vi "ISO226.vi"(11 "Phone number":dbl=1.0) -> (2 "SPL":dbl[](array[numeric]), 3 "Frequency":dbl[](array[numeric]))   [LabVIEW 2013]
uses:
  Stimulus/SubVI/CRYStimulus Global.vi
panel:
  out "XY Graph":cluster{dbl[], dbl[]}(graph)
  out "f":dbl[](array[numeric])
  in  "step number":i32=29
  in  "Resolution":u16
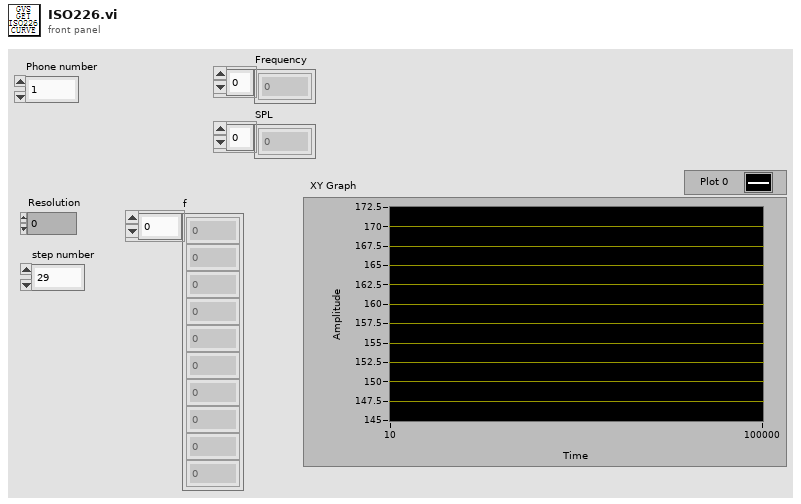
[diagram p1: front panel]
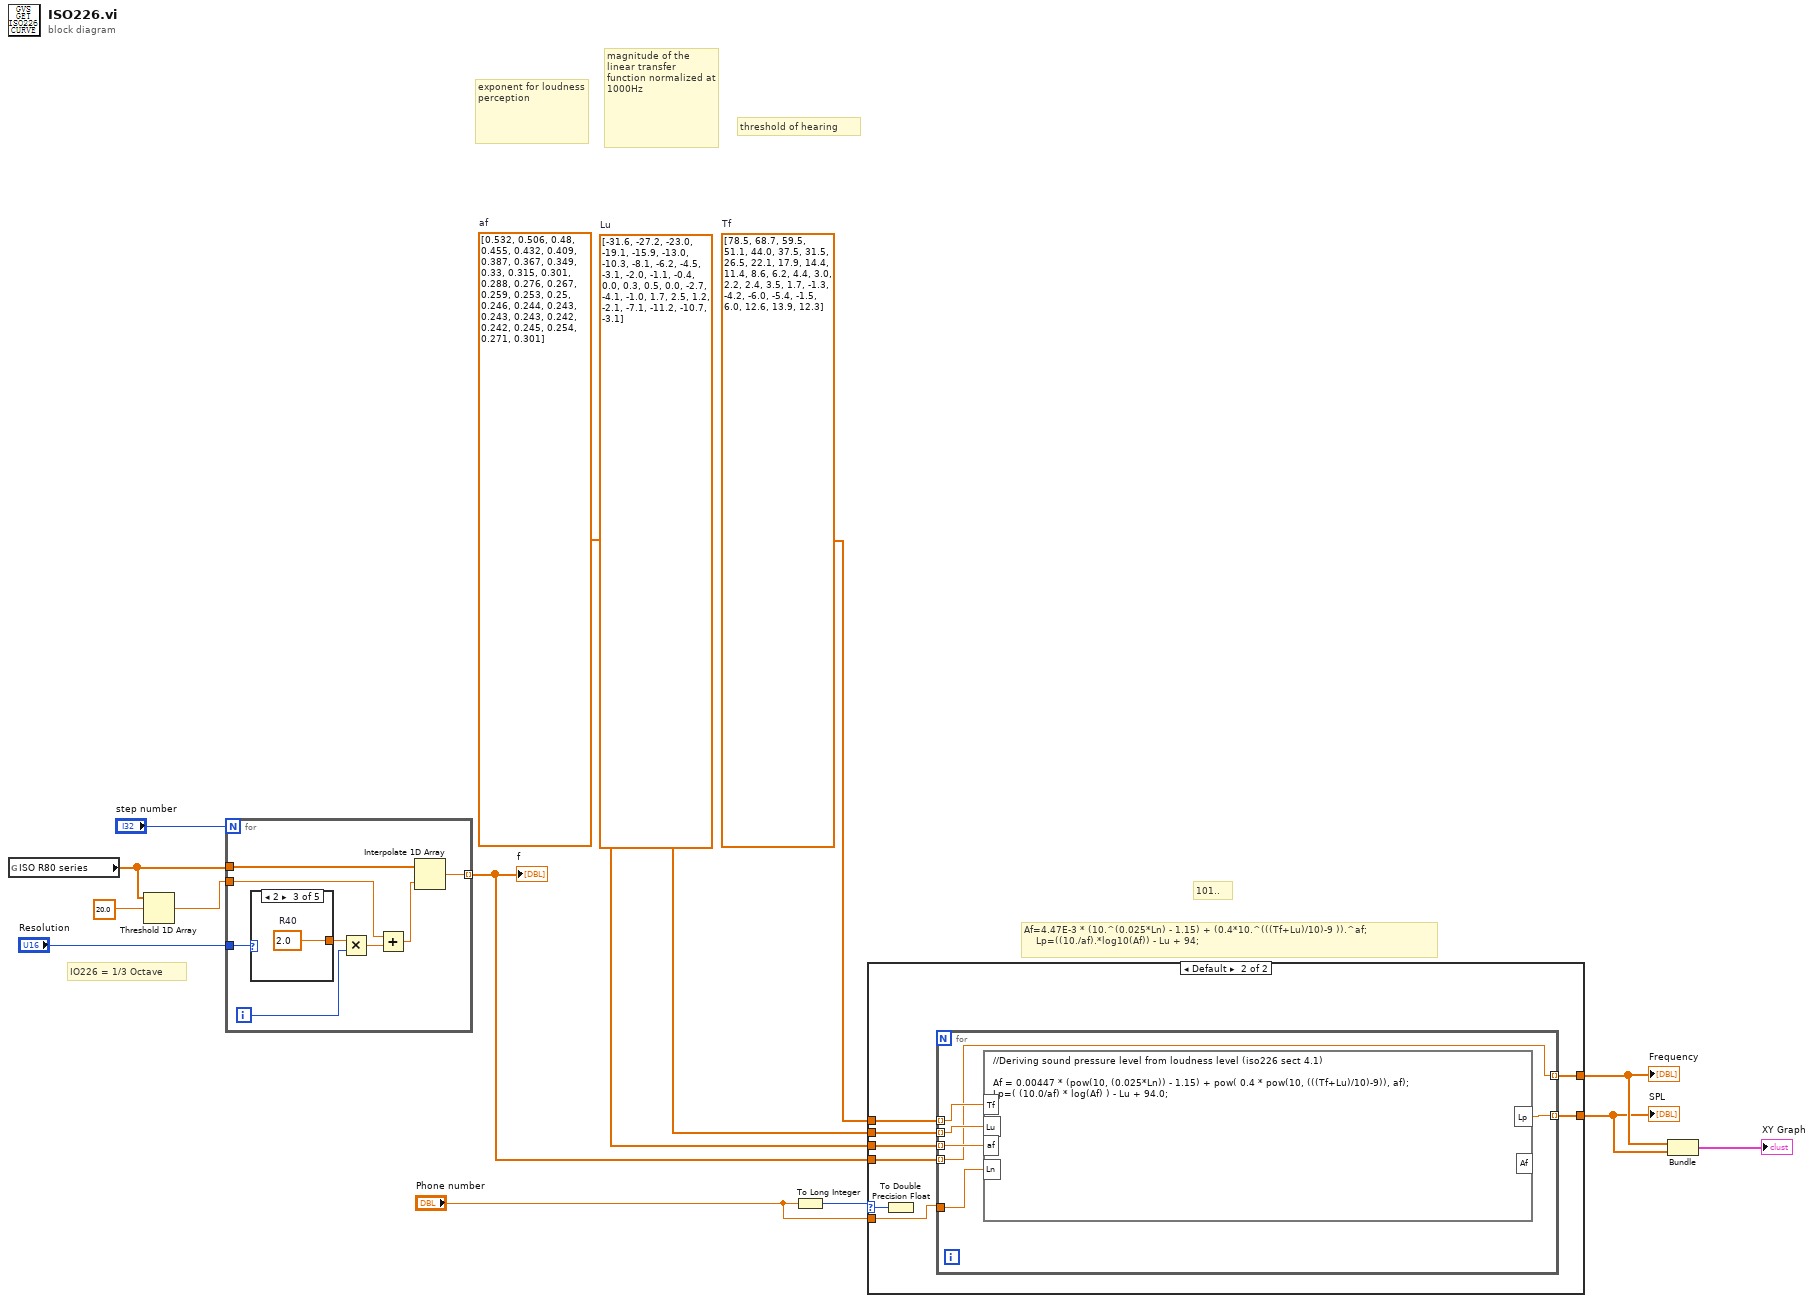
[diagram p0: block diagram]
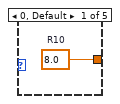
[diagram p3: hidden frame]
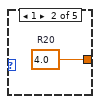
[diagram p4: hidden frame]
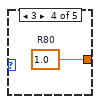
[diagram p5: hidden frame]
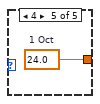
[diagram p6: hidden frame]
diagram:
  w4 = dbl[] [78.5, 68.7, 59.5, 51.1, 44.0, 37.5, 31.5, 26.5, 22.1, 17.9, 14.4, 11.4, 8.6, 6.2, 4.4, 3.0, 2.2, 2.4, 3.5, 1.7, -1.3, -4.2, -6.0, -5.4, -1.5, 6.0, 12.6, 13.9, 12.3]  # Tf
  w3 = dbl[] [-31.6, -27.2, -23.0, -19.1, -15.9, -13.0, -10.3, -8.1, -6.2, -4.5, -3.1, -2.0, -1.1, -0.4, 0.0, 0.3, 0.5, 0.0, -2.7, -4.1, -1.0, 1.7, 2.5, 1.2, -2.1, -7.1, -11.2, -10.7, -3.1]  # Lu
  w10 = dbl[] [0.532, 0.506, 0.48, 0.455, 0.432, 0.409, 0.387, 0.367, 0.349, 0.33, 0.315, 0.301, 0.288, 0.276, 0.267, 0.259, 0.253, 0.25, 0.246, 0.244, 0.243, 0.243, 0.243, 0.242, 0.242, 0.245, 0.254, 0.271, 0.301]  # af
  # "101.."
  # "IO226 = 1/3 Octave"
  # "Af=4.47E-3 * (10.^(0.025*Ln) - 1.15) + (0.4*10.^(((Tf+Lu)/10)-9 )).^af;\n    Lp=((10./af).*log10(Af)) - Lu + 94;"
  # "threshold of hearing"
  # "magnitude of the linear transfer\nfunction normalized at 1000Hz"
  # "exponent for loudness perception"
  n1 = global read "CRYStimulus Global.vi" "ISO R80 series"() -> (w1:dbl[])
  n2 = Threshold 1D Array(2:20.0 ("x*y"), 3:w1) -> (0:w12:dbl)  [unwired: 1 out]
  n3 = for {
    N: "step number" -> [_]
    tunnel: w1 -> [w21]
    tunnel: [w19] -> w5 mode=indexing
    tunnel: "Resolution" -> [w18]
    tunnel: w12 -> [w16]
    i -> [w20]
    n4 = case shown="2" w18 {
      tunnel: [w23 w24 w25 w26 w27] -> w22
      frame 0, Default {
        w23 = 8.0  # R10
      }
      frame 1 {
        w24 = 4.0  # R20
      }
      frame 2 {
        w25 = 2.0  # R40
      }
      frame 3 {
        w26 = 1.0  # R80
      }
      frame 4 {
        w27 = 24.0  # 1 Oct
      }
    }
    n5 = Multiply(x=w22, y=w20) -> (x*y=w17:dbl)
    n6 = Add(x=w16, y=w17) -> (x+y=w15:dbl)
    n7 = Interpolate 1D Array(1:w15, 2:w21) -> (0:w19:dbl)
  }
  "f" <- w5
  n8 = To Long Integer(number="Phone number") -> (32bit integer=w7:i32)
  n9 = case shown="Default" w7 {
    selector: w7 -> [_ w35]
    tunnel: w5 -> [_ w28]
    tunnel: w4 -> [_ w31]
    tunnel: w3 -> [_ w30]
    tunnel: w10 -> [_ w29]
    tunnel: [_ w33] -> w9
    tunnel: [_ w34] -> w2
    tunnel: "Phone number" -> [_ w32]
    frame ..-1 {
    }
    frame Default {
      n10 = To Double Precision Float(number=w35) -> ()  [unwired: 1 out]
      n11 = for {
        tunnel: w28 -> [w36] mode=indexing
        tunnel: w32 -> [w41]
        tunnel: [w40] -> w34 mode=indexing
        tunnel: w31 -> [w37] mode=indexing
        tunnel: w30 -> [w38] mode=indexing
        tunnel: w29 -> [w39] mode=indexing
        tunnel: [w36] -> w33 mode=indexing
        n12 = formula code="//Deriving sound pressure level from loudness level (iso226 sect 4.1)\n\nAf = 0.00447 * (pow(10, (0.025*Ln)) - 1.15) + pow( 0.4 * pow(10, (((Tf+Lu)/10)-9)), af);\nLp=( (10.0/af) * log(Af) ) - Lu + 94.0;"("Ln"=w41, "Tf"=w37, "Lu"=w38, "af"=w39) -> ("Lp"=w40:dbl)  [unwired: 1 out]
      }
    }
  }
  "Frequency" <- w9
  "SPL" <- w2
  n13 = Bundle(w9, w2) -> (→"XY Graph":cluster{dbl[], dbl[]})  [unwired: 1 in]
